vi "PluginSearchPath_Test.vi"() -> ()   [LabVIEW 2021]
uses:
  labbCAN_Bus_API/labbCAN_Bus_API.lvlib
panel:
  out "error out":errorcluster caption="Fehler (Ausgang)"
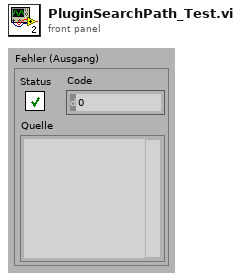
[diagram p1: front panel]
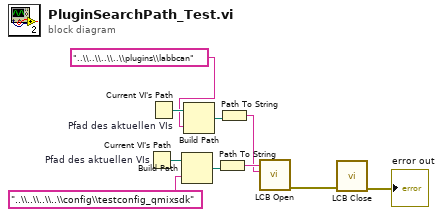
[diagram p0: block diagram]
diagram:
  n1 = Current VI's Path "Pfad des aktuellen VIs"() -> (path=w9:path)
  n2 = Current VI's Path "Pfad des aktuellen VIs"() -> (path=w6:path)
  n3 = Build Path(base path=w9, name or relative path="..\\..\\..\\..\\config\\testconfig_qmixsdk" ("Name oder relativer Pfad")) -> (appended path=w7:path)
  n4 = Build Path(base path=w6, name or relative path="..\\..\\..\\..\\plugins\\labbcan" ("Name oder relativer Pfad")) -> (appended path=w5:path)
  n5 = Path To String(path=w7) -> (string=w10:string)
  n6 = Path To String(path=w5) -> (string=w4:string)
  n7 = call "LCB Open.vi"("PluginSearchPath"=w4, "Device Configuration Path"=w10) -> ("error out"=w2:errorcluster)  [unwired: 9 in]
  n8 = call "LCB Close.vi"("error in (no error)"=w2) -> ("error out"=→"error out":errorcluster)  [unwired: 10 in]
